vi "Check.vi"(7 "Address":string, 8 "Error In":errorcluster) -> (0 "Error Out":errorcluster)   [LabVIEW 2018, in "Tests.lvlib" / "KnownHosts.lvlib"]
uses:
  KnownHosts.lvlib
  src/Toolkit/API/Known Hosts/API/Typedefs/Check Results.ctl
  <vilib>/Utility/error.llb/Clear Errors.vi
  <vilib>/Utility/file.llb/Is Path and Not Empty.vi
  <vilib>/Utility/sysdir.llb/Get System Directory.vi
  <vilib>/addons/_JKI Toolkits/Caraya/classes/Test/Test.lvclass
  <vilib>/addons/_JKI Toolkits/Caraya/classes/Assert/Assert.lvclass
  src/Toolkit/API/Known Hosts/Known Hosts.lvclass
  Tests.lvlib
  src/Toolkit/API/Session/Session.lvclass
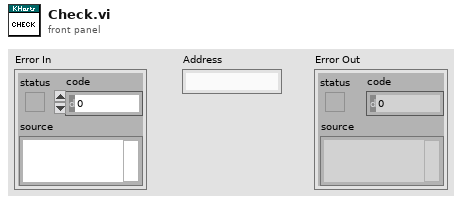
[diagram p1: front panel]
types:
  T1 = typedef "Toolkit.lvlib/Known Hosts.lvclass/Check Results.ctl" = enum32{"Failure", "Mismatch", "Match", "Not Found"}
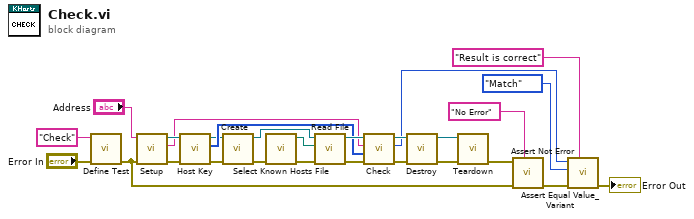
[diagram p0: block diagram]
diagram:
  n1 = call <vilib>:"Define Test.vi"("error in (no error)"="Error In", "Label (VI Title)"="Check") -> ("error out"=w7:errorcluster)  [unwired: 9 in]
  n2 = call "Setup.vi"("Error In"=w7, "Address In"="Address") -> ("Error Out"=w8:errorcluster, "Address Out"=w5:string, "Sesssion"=w9:refnum<class "Session.lvclass">)  [unwired: 7 in]
  n3 = call "Host Key.vi"("Error In"=w8, "Session In"=w9) -> ("Error Out"=w11:errorcluster, "Host Key"=w10:u8[], "Sesssion Out"=w4:refnum<class "Session.lvclass">)  [unwired: 6 in, 1 out]
  n4 = call "Create.vi"("Error In"=w11, "Session"=w4) -> ("Error Out"=w23:errorcluster, "Known Hosts"=w24:refnum<class "Known Hosts.lvclass">)  [unwired: 8 in]
  n5 = call "Select Known Hosts File.vi"("Error In"=w23) -> ("Error Out"=w22:errorcluster, "Known Hosts File"=w21:path)  [unwired: 9 in]
  n6 = call "Read File.vi"("Error In"=w22, "File"=w21, "KnownHosts In"=w24) -> ("Error Out"=w13:errorcluster, "KnownHosts Out"=w19:refnum<class "Known Hosts.lvclass">)  [unwired: 6 in, 1 out]
  n7 = call "Check.vi"("Error In"=w13, "Host Key"=w10, "Address"=w5, "KnownHosts In"=w19) -> ("Error Out"=w14:errorcluster, "Result"=w12:T1, "KnownHosts Out"=w18:refnum<class "Known Hosts.lvclass">)  [unwired: 5 in]
  n8 = call "Destroy.vi"("Error In"=w14, "KnownHosts"=w18) -> ("Error Out"=w3:errorcluster, "Session"=w1:refnum<class "Session.lvclass">)  [unwired: 8 in]
  n9 = call "Teardown.vi"("Error In"=w3, "Session"=w1) -> ("Error Out"=w2:errorcluster)  [unwired: 9 in]
  n10 = call <vilib>:"Assert Not Error.vi"("Label"="No Error", "error in (no error)"=w7, "Not Error?"=w2) -> ("error out"=w20:errorcluster)  [unwired: 8 in]
  n11 = call <vilib>:"Assert Equal Value_Variant.vi"("Label"="Result is correct", "error in (no error)"=w20, "Y"=Check_Results."Match" ("Result"), "X"=w12) -> ("error out"=→"Error Out":errorcluster)  [unwired: 7 in]
